vi "analyseData.vi"(8 "error in (no error)":errorcluster, 10 "HGF_VariantDataObject in":refnum<class "HGF_VariantDataObject.lvclass">, 11 "HGF_DataAnalysator in":refnum<class "HGF_DataAnalysator.lvclass">) -> (0 "error out":errorcluster, 2 "HGF_VariantDataObject out":refnum<class "HGF_VariantDataObject.lvclass">, 3 "HGF_DataAnalysator out":refnum<class "HGF_DataAnalysator.lvclass">)   [LabVIEW 2012, in "HGF_DataAnalyzer.lvlib" / "HGF_DataAnalysator.lvclass"]
doc: "Analyse data contained in HGF_DataVariantObject.\n\nThis is a dynamic dispatch VI to be overwritten by child classes."
uses:
  HGF_DataAnalysator.lvclass
  HGF_LVC/HGF_BaseClasses/HGF_VariantDataObject/HGF_VariantDataObject.lvclass
  HGF_DataAnalysis/HGF_DataAnalysis.lvclass
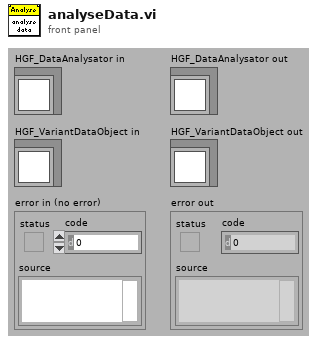
[diagram p1: front panel]
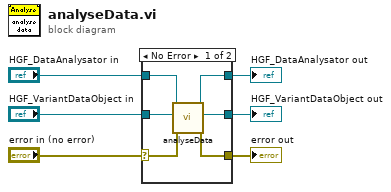
[diagram p0: block diagram]
diagram:
  n1 = case shown="No Error" "error in (no error)" {
    selector: "error in (no error)" -> [w9 w15]
    tunnel: [w8 w15] -> w5
    tunnel: [w11 w14] -> w3
    tunnel: "HGF_DataAnalysator in" -> [w12 w14]
    tunnel: [w7 w13] -> w2
    tunnel: "HGF_VariantDataObject in" -> [w10 w13]
    frame No Error {
      n2 = call-parent "analyseData.vi"("error in (no error)"=w9, "HGF_VariantDataObject in"=w10, "HGF_DataAnalysis in"=w12) -> ("error out"=w8:errorcluster, "HGF_VariantDataObject out"=w7:refnum<class "HGF_VariantDataObject.lvclass">, "HGF_DataAnalysis out"=w11:refnum<class "HGF_DataAnalysator.lvclass">)  [unwired: 6 in]
    }
    frame Error {
    }
  }
  "error out" <- w5
  "HGF_DataAnalysator out" <- w3
  "HGF_VariantDataObject out" <- w2
